vi "Close Config File.vi"(8 "error in (no error)":errorcluster, 11 "Configuration File In":refnum<class "Configuration.lvclass">) -> (0 "error out":errorcluster, 2 "file path":path, 3 "Configuration File Out":refnum<class "Configuration.lvclass">)   [LabVIEW 2020, in "Configuration.lvclass"]
doc: "High-level function for opening configuration file data from Process class."
uses:
  Configuration.lvclass
  <vilib>/Utility/config.llb/NI_LVConfig.lvlib
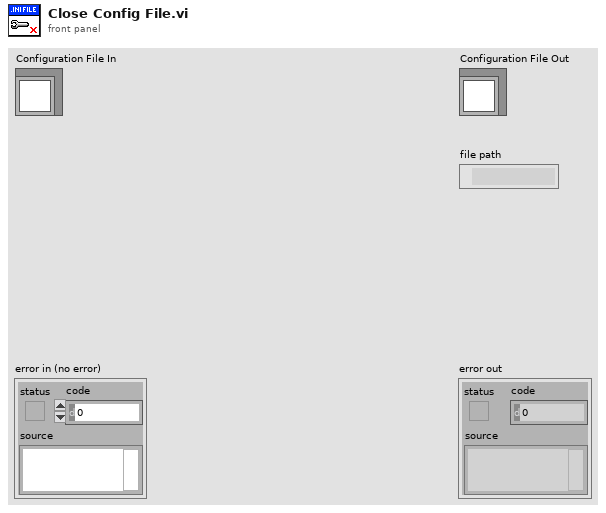
[diagram p1: front panel]
types:
  T1 = typedef "NI_LVConfig.lvlib/Config Data RefNum.ctl" = refnum<k1>
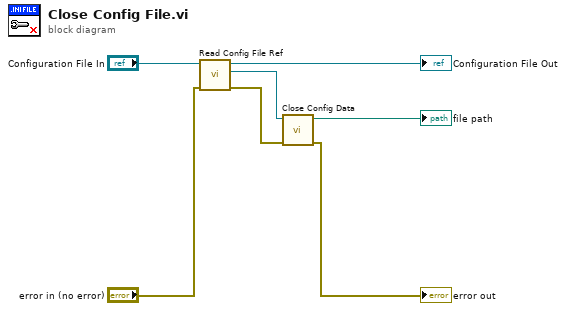
[diagram p0: block diagram]
diagram:
  n1 = call-dynamic "Read Config File Ref.vi"("error in (no error)"="error in (no error)", "Configuration File In"="Configuration File In") -> ("error out"=w2:errorcluster, "refnum out"=w3:T1, "Configuration File Out"=→"Configuration File Out":refnum<class "Configuration.lvclass">)  [unwired: 7 in]
  n2 = call <vilib>:"Close Config Data.vi"("error in (no error)"=w2, "refnum"=w3) -> ("error out"=→"error out":errorcluster, "file path"=→"file path":path)  [unwired: 8 in]
